vi "Actor Core.vi"(8 "error in":errorcluster, 11 "Camera in":refnum<class "Camera.lvclass">) -> (0 "error out":errorcluster, 3 "Actor out":refnum<class "Actor.lvclass">)   [LabVIEW 2023, in "Camera.lvlib" / "Camera.lvclass"]
doc: "(<B>Filename</B>: Actor Framework.lvlib:Actor.lvclass:Actor Core.vi)\n\nReceives messages to the actor, reacts to them, and initiates any error handling that may shut the actor down.\n\nDescendant classes may override this VI to append parallel tasks for the actor to complete while it handles messages. Overrides use the Call Parent Method node."
uses:
  Camera.lvclass
  Camera.lvclass/Camera.ctl
  <vilib>/ActorFramework/Actor/Actor.lvclass
  <vilib>/ActorFramework/Message Enqueuer/Message Priority.ctl
  <vilib>/ActorFramework/Message Enqueuer/Message Enqueuer.lvclass
  Camera Messages/Get Most Recent Frame (if active) Msg/Get Most Recent Frame (if active) Msg.lvclass
  Resources/GLOBAL/GLOBAL Time-critical.vi
  C:/FlashGordon/Development/Hardware/Device/Device.lvclass
  C:/Program Files/National Instruments/LabVIEW 2023/vi.lib/ActorFramework/Actor/Actor.lvclass
  C:/FlashGordon/Development/Hardware/Camera/Camera.lvclass
  Tiff Writer/Tiff Writer/Tiff Writer.lvclass
  Device/Device.lvclass
  C:/FlashGordon/Development/Hardware/Tiff Writer/Tiff Writer/Tiff Writer.lvclass
panel:
  in  "Stop Button":bool
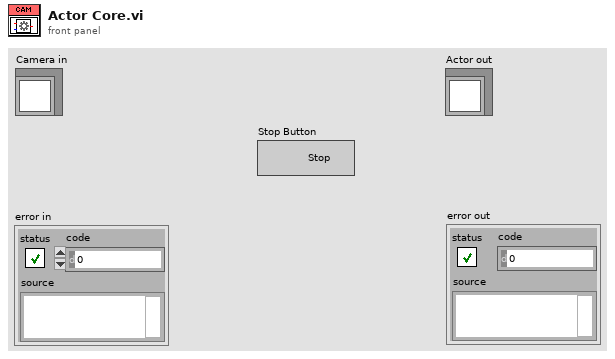
[diagram p1: front panel]
types:
  T1 = typedef "Actor Framework.lvlib/Message Enqueuer.lvclass/Message Priority.ctl" = enum16{"Low", "Normal", "High"}
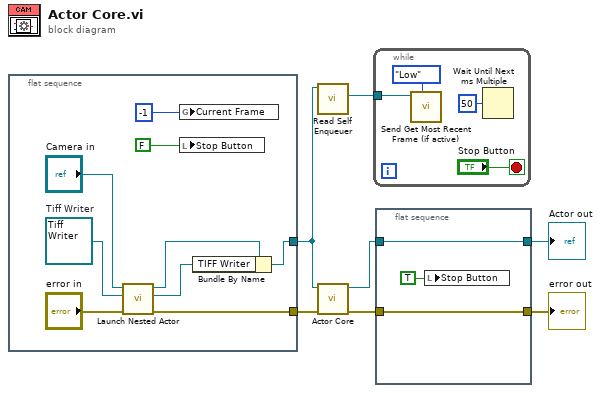
[diagram p0: block diagram]
diagram:
  n1 = flat-sequence {
    tunnel: [w11] -> w7
    tunnel: [w14] -> w2
    frame #0 {
      w9 = refnum<class "Tiff Writer.lvclass"> refnum  # Tiff Writer
      n2 = call <vilib>:"Launch Nested Actor.vi"("error in (no error)"="error in", "Nested Actor"=w9, "Caller Actor in"="Camera in") -> ("error out"=w11:errorcluster, "Nested Actor's Enqueuer"=w13:refnum<class "Message Enqueuer.lvclass">, "Caller Actor out"=w8:refnum<class "Camera.lvclass">)  [unwired: 6 in]
      n3 = global write "GLOBAL Time-critical.vi" "Current Frame"(-1 ("Current Frame")) -> ()
      n4 = local write "Stop Button"(FALSE ("Stop Button")) -> ()
      n5 = Bundle By Name(cluster=w8, "TIFF Writer"=w13) -> (w14:refnum<class "Camera.lvclass">)
    }
  }
  n6 = call <vilib>:"Read Self Enqueuer.vi"("Actor"=w2) -> ("Self Enqueuer"=w6:refnum<class "Message Enqueuer.lvclass">)  [unwired: 10 in]
  n7 = call-parent "Actor Core.vi"("error in"=w7, "Device in"=w2) -> ("error out"=w4:errorcluster, "Actor out"=w1:refnum<class "Actor.lvclass">)  [unwired: 8 in]
  n8 = while {
    tunnel: w6 -> [w17]
    stop <- "Stop Button" stop-if-true
    n9 = call "Send Get Most Recent Frame (if active).vi"("Message Priority (Normal)"=Message_Priority."Low", "Message Enqueuer"=w17) -> ()  [unwired: 8 in, 2 out]
    n10 = Wait Until Next ms Multiple(millisecond multiple=u32 50) -> ()  [unwired: 1 out]
  }
  n11 = flat-sequence {
    tunnel: [w23] -> w5
    tunnel: w1 -> [w23]
    tunnel: w4 -> [w22]
    tunnel: [w22] -> w3
    frame #0 {
      n12 = local write "Stop Button"(TRUE ("Stop Button")) -> ()
    }
  }
  "error out" <- w3
  "Actor out" <- w5
